vi "accept.vi"(8 "error in (no error)":errorcluster, 10 "Visitor":refnum<class "Visitor.lvclass">, 11 "Dot in":refnum<class "Dot.lvclass">) -> (0 "error out":errorcluster, 2 "String":string, 3 "Dot out":refnum<class "Dot.lvclass">)   [LabVIEW 2018, in "Dot.lvclass"]
uses:
  Dot.lvclass
  Visitor Class/Visitor.lvclass
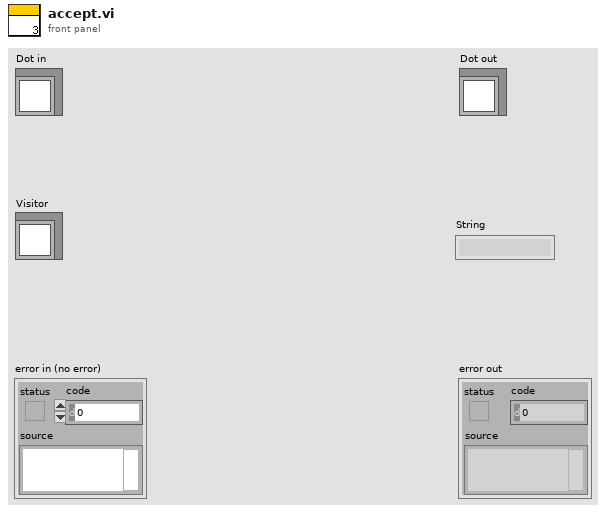
[diagram p1: front panel]
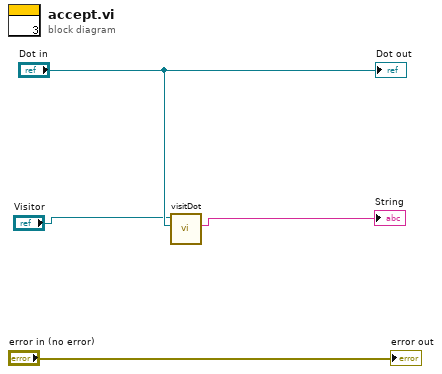
[diagram p0: block diagram]
diagram:
  n1 = call-dynamic "visitDot.vi"("Dot"="Dot in", "Visitor in"="Visitor") -> ("String"=→"String":string)  [unwired: 7 in, 2 out]
  "error out" <- "error in (no error)"
  "Dot out" <- "Dot in"
